vi "2D_Plot.ly_multi_Ex.vi"() -> ()   [LabVIEW 2025]
doc: "Demonstratese how to plot an array with timebase to Plot.ly."
uses:
  <vilib>/Foerster.tech/LabPlot.ly/LabPlot.ly/Typdef/graphSettings.ctl
  <vilib>/Foerster.tech/LabPlot.ly/LabPlot.ly/Typdef/mode.ctl
  <vilib>/Foerster.tech/LabPlot.ly/LabPlot.ly/Typdef/line.ctl
  <vilib>/Foerster.tech/LabPlot.ly/LabPlot.ly/Typdef/dash.ctl
  <vilib>/Analysis/1siggen.llb/Ramp Pattern by Samples.vi
  <vilib>/Analysis/NI_AALBase.lvlib
  <vilib>/Foerster.tech/LabPlot.ly/LabPlot.ly/LabPlot.ly.lvlib
panel:
  in  "Samples[]":i32[](array[numeric])=[50000, 25, 250]
  in  "Reduction[]":i32[](array[numeric])=[0, 0, 0]
  in  "graphSettings[]":T1[](array[typedef])=[{"mode"=enum."lines", "line"={"color"=44543, "width"=1, "dash"=enum."dashdot"}}, {"mode"=enum."lines+markers", "line"={"color"=13816530, "width"=1, "dash"=enum."solid"}}, {"mode"=enum."lines+markers", "line"={"color"=16760338, "width"=1, "dash"=enum."dash"}}]
  out "File Path out":path
  out "Execution Time[ms]":u32
  in  "cycles":dbl=5.0 format="%0.2f"
  in  "Call Setup":bool
  in  "File Path Control(empty: only show graph)":path
  in  "amplitude":dbl=5.0 format="%0.2f"
  out "XY Graph":T5(graph)
  # "Sinewave Settings"
  # "Call asynchronously to not hold up your program"
  # "This Program demonstrates how to print multiple 2D Array consisting of timebase and data to Plot.ly\n\nYou can output the plot to browser without saving it by leaving File Path empty or save the html file by selecting a path.\n\nSince Plot.ly stores the data in the html, plots of >200k points become slow to open. It's recommended you use the built-in Reduction to reduce your dataset."
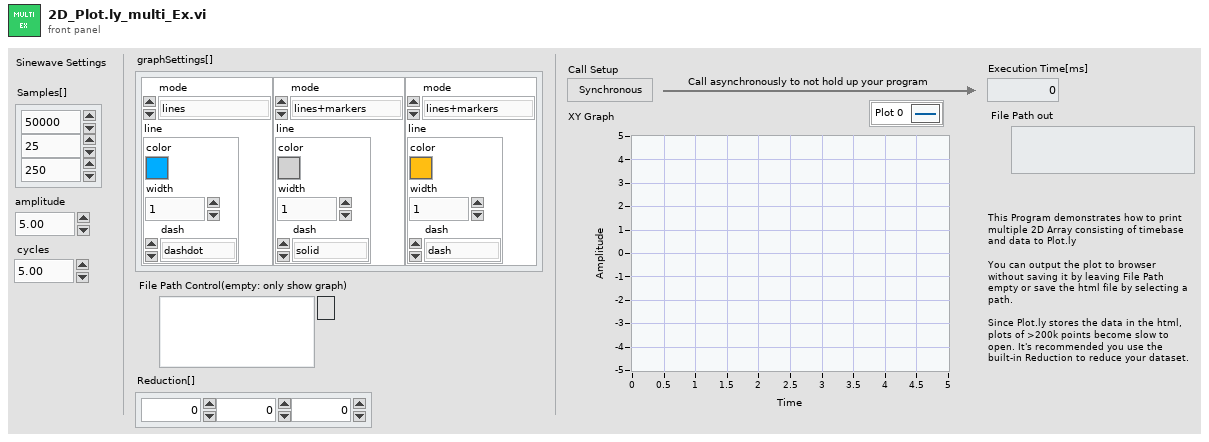
[diagram p1: front panel]
types:
  T1 = typedef "LabPlot.ly.lvlib/graphSettings.ctl" = cluster{"mode":T2, "line":T3}
  T2 = typedef "LabPlot.ly.lvlib/mode.ctl" = enum16{"lines", "markers", "text", "lines+markers", "markers+text", "lines+text", "lines+markers+text"}
  T3 = typedef "LabPlot.ly.lvlib/line.ctl" = cluster{"color":u32, "width":i32, "dash":T4}
  T4 = typedef "LabPlot.ly.lvlib/dash.ctl" = enum16{"solid", "dot", "dash", "longdash", "dashdot", "longdashdot"}
  T5 = cluster{"Ramp Pattern":dbl[], "Sinusoidal Pattern":dbl[]}[]
  T6 = cluster{"Ramp Pattern":dbl[], "Sinusoidal Pattern":dbl[]}
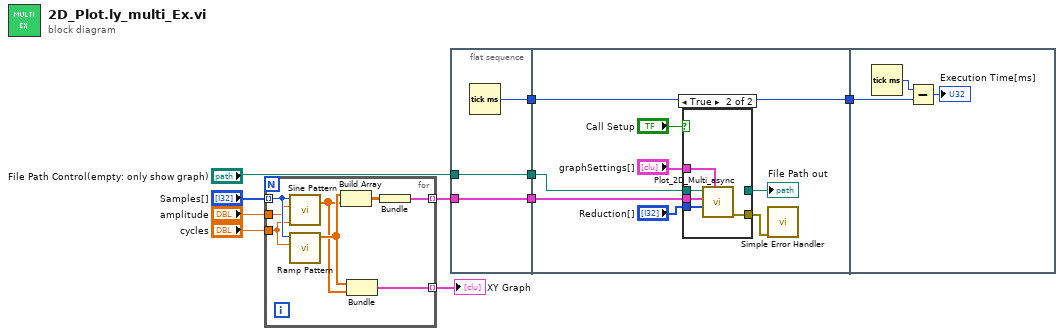
[diagram p0: block diagram]
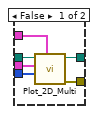
[diagram p2: hidden frame]
diagram:
  n1 = for {
    tunnel: "Samples[]" -> [w15] mode=indexing
    tunnel: "amplitude" -> [w14]
    tunnel: "cycles" -> [w13]
    tunnel: [w12] -> w2 mode=indexing
    tunnel: [w11] -> w1 mode=indexing
    n2 = call <vilib>:"Sine Pattern.vi"("cycles"=w13, "amplitude"=w14, "samples"=w15) -> ("Sinusoidal Pattern"=w16:dbl[])  [unwired: 1 in, 1 out]
    n3 = call-poly <vilib>:"Ramp Pattern.vi"("end"=w13, "samples"=w15) -> ("Ramp Pattern"=w17:dbl[])  [unwired: 8 in, 1 out]
    n4 = Build Array(w17, w16) -> (w18:dbl[][])
    n5 = Bundle("Ramp Pattern"=w17, "Sinusoidal Pattern"=w16) -> (w11:T6)  [unwired: 1 in]
    n6 = Bundle(w18) -> (w12:cluster{dbl[][]})  [unwired: 1 in]
  }
  "XY Graph" <- w1
  n7 = flat-sequence {
    tunnel: "File Path Control(empty: only show graph)" -> [w21]
    tunnel: [w21] -> w10
    tunnel: [w20] -> w9
    tunnel: w2 -> [w19]
    tunnel: [w19] -> w7
    tunnel: w10 -> [w29]
    tunnel: w9 -> [w28]
    tunnel: [w28] -> w8
    tunnel: w7 -> [w27]
    tunnel: w8 -> [w42]
    frame #0 {
      n8 = Tick Count (ms)() -> (millisecond timer value=w20:u32)
    }
    frame #1 {
      n9 = case shown="True" "Call Setup" {
        tunnel: "Reduction[]" -> [w35 w38]
        tunnel: w29 -> [w34 w40]
        tunnel: "graphSettings[]" -> [w30 w39]
        tunnel: [w33 w37] -> w25
        tunnel: [w32 _] -> w26
        tunnel: w27 -> [w31 w36]
        frame False {
          n10 = call <vilib>:"Plot_2D_Multi.vi"("graphSettings[]"=w30, "Reduction(0: No Reduction)"=w35, "2D-Data[]"=w31, "File Path Control(empty: only show graph)"=w34) -> ("Error Out"=w33:errorcluster, "File Path Indicator"=w32:path)  [unwired: 6 in]
        }
        frame True {
          n11 = call <vilib>:"Plot_2D_Multi_async.vi"("graphSettings[]"=w39, "Reduction(0: No Reduction)"=w38, "2D-Data[]"=w36, "File Path Control(empty: only show graph)"=w40) -> ("Error Out"=w37:errorcluster)  [unwired: 7 in]
        }
      }
      "File Path out" <- w26
      n12 = call <vilib>:"Simple Error Handler.vi"("error in (no error)"=w25) -> ()  [unwired: 4 in, 5 out]
    }
    frame #2 {
      n13 = Tick Count (ms)() -> (millisecond timer value=w43:u32)
      n14 = Subtract(x=w43, y=w42) -> (x-y=→"Execution Time[ms]":u32)
    }
  }
